vi "Register for Broadcast Events.vi"(8 "error in (no error)":errorcluster, 11 "Application In":refnum<class "Application.lvclass">) -> (0 "error out":errorcluster, 2 "Event Registration Refnum":refnum<event-registration>, 3 "Application Out":refnum<class "Application.lvclass">)   [LabVIEW 2020, in "Application.lvclass"]
doc: "Get a registration for broadcast events for the application and all owned processes."
uses:
  Application.lvclass
  Process/Protected/Broadcasting/Broadcast Message Cluster.ctl
  Process/Process.lvclass
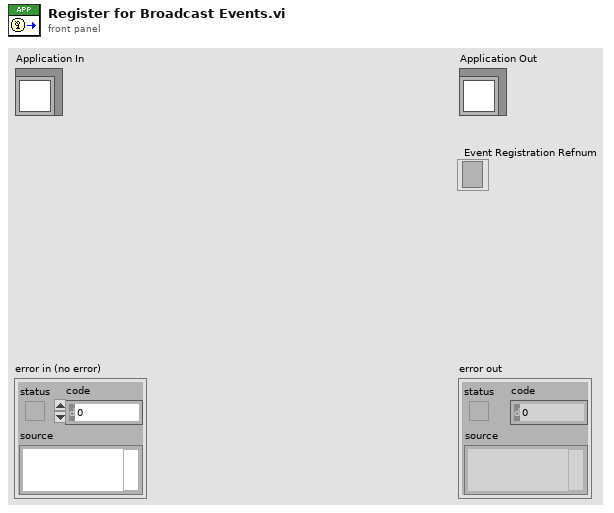
[diagram p1: front panel]
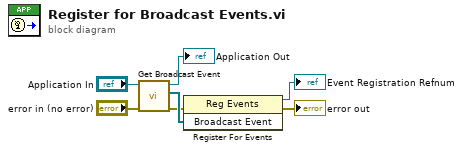
[diagram p0: block diagram]
diagram:
  n1 = call-dynamic "Get Broadcast Event.vi"("error in (no error)"="error in (no error)", "Application in"="Application In") -> ("error out"=w2:errorcluster, "Broadcast Event"=w4:refnum<user-event>[], "Application out"=→"Application Out":refnum<class "Application.lvclass">)  [unwired: 7 in]
  n2 = register-events(error in=w2, w4) -> (reference out=→"Event Registration Refnum":refnum<event-registration>, error out=→"error out":errorcluster)  [unwired: 1 in]
